vi "2 WaypointHeadingGoodness.vi"(3 "Waypoint Location":T1 {"North" format="%#_10f"; "East" format="%#_8f"}, 4 "Heading to Test":dbl) -> (1 "Goodness":dbl)   [LabVIEW 2011]
doc: "Takes the absolute wind vector, the heading of your next waypoint, and a test heading and outputs a goodness value for the test heading. The criteria is the speed to get to the waypoint.\n\nThe goodness is evaluated by taking the softmax of an angle with all possible complimenting angles (i.e. if the test heading is 10 degrees it is matched with -1 through -89; note that angles are adjusted to be degrees from directly at the waypoint). The specific calculation for finding the net velocity of a pair of angles requires the velocities from the polar plot."
uses:
  2 Typedefs/UTM Location.ctl
  2 Globals/2 Global.vi
  2 Globals/2 TuningConstants.vi
panel:
  out "Heading to Waypt":dbl
  # "Inputs"
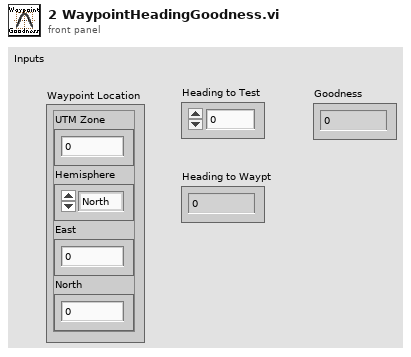
[diagram p1: front panel]
types:
  T1 = typedef "UTM Location.ctl" = cluster{"UTM Zone":dbl, "Hemisphere":enum16{"North", "South"}, "East":dbl, "North":dbl}
  T2 = typedef "Velocity.ctl" = cluster{"East":dbl, "North":dbl}
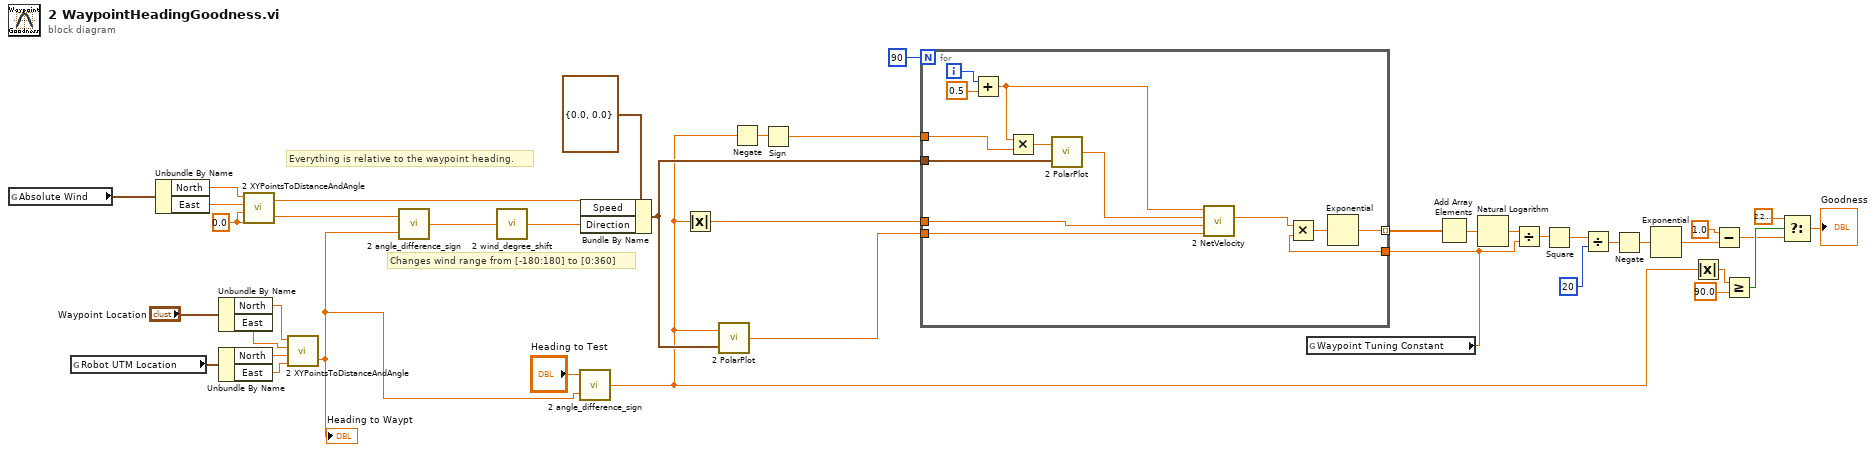
[diagram p0: block diagram]
diagram:
  w8 = 0.0
  # "Changes wind range from [-180:180] to [0:360]"
  # "Everything is relative to the waypoint heading."
  n1 = global read "2 Global.vi" "Absolute Wind"() -> (w11:T2)
  n2 = global read "2 Global.vi" "Robot UTM Location"() -> (w12:T1)
  n3 = Unbundle By Name(w11) -> ("North"=w9:dbl, "East"=w10:dbl)
  n4 = Unbundle By Name("Waypoint Location") -> ("North"=w21:dbl, "East"=w20:dbl)
  n5 = Unbundle By Name(w12) -> ("North"=w22:dbl, "East"=w23:dbl)
  n6 = call "2 XYPointsToDistanceAndAngle.vi"("East 2"=w8, "North 2"=w8, "East 1"=w10, "North 1"=w9) -> ("Angle Diff"=w25:dbl, "Distance"=w24:dbl)
  n7 = call "2 XYPointsToDistanceAndAngle.vi"("East 2"=w23, "North 2"=w22, "East 1"=w20, "North 1"=w21) -> ("Angle Diff"=w37:dbl)  [unwired: 1 out]
  "Heading to Waypt" <- w37
  n8 = call "2 angle_difference_sign.vi"("Angle 2"=w37, "Angle 1"=w25) -> ("Difference"=w41:dbl)
  n9 = call "2 wind_degree_shift.vi"("Wind Theta -180 - 180"=w41) -> ("Wind Theta 0-360"=w40:dbl)
  n10 = call "2 angle_difference_sign.vi"("Angle 2"=w37, "Angle 1"="Heading to Test") -> ("Difference"=w4:dbl)
  n11 = Bundle By Name(cluster=cluster{"Speed":dbl, "Direction":dbl} {"Speed"=0.0, "Direction"=0.0} ("input cluster"), "Speed"=w24, "Direction"=w40) -> (w27:cluster{"Speed":dbl, "Direction":dbl})
  n12 = Absolute Value(x=w4) -> (abs(x)=w2:dbl)
  n13 = call "2 PolarPlot.vi"("Wind Vector"=w27, "Boat Angle"=w4) -> ("Velocity"=w1:dbl)
  n14 = Negate(x=w4) -> (-x=w5:dbl)
  n15 = Sign(1:w5) -> (0:w6:dbl)
  n16 = global read "2 TuningConstants.vi" "Waypoint Tuning Constant"() -> (w3:dbl)
  n17 = for {
    N: 90 -> [_]
    tunnel: w27 -> [w54]
    tunnel: [w50] -> w13 mode=indexing
    tunnel: w6 -> [w43]
    tunnel: w3 -> [w45]
    tunnel: w2 -> [w47]
    tunnel: w1 -> [w46]
    i -> [w52]
    n18 = Add(x=w52, y=0.5) -> (x+y=w42:dbl)
    n19 = Multiply(x=w42, y=w43) -> (x*y=w53:dbl)
    n20 = call "2 PolarPlot.vi"("Wind Vector"=w54, "Boat Angle"=w53) -> ("Velocity"=w48:dbl)
    n21 = call "2 NetVelocity.vi"("Speed 2"=w46, "Angle 2"=w47, "Speed 1"=w48, "Angle 1"=w42) -> ("Net Velocity"=w44:dbl)  [unwired: 7 in]
    n22 = Multiply(x=w44, y=w45) -> (x*y=w49:dbl)
    n23 = Exponential(1:w49) -> (0:w50:dbl)
  }
  n24 = Add Array Elements(numeric array=w13) -> (sum=w16:dbl)
  n25 = Natural Logarithm(1:w16) -> (0:w15:dbl)
  n26 = Divide(x=w15, y=w3) -> (x/y=w14:dbl)
  n27 = Square(x=w14) -> (x^2=w17:dbl)
  n28 = Divide(x=w17, y=20) -> (x/y=w18:dbl)
  n29 = Negate(x=w18) -> (-x=w29:dbl)
  n30 = Exponential(1:w29) -> (0:w30:dbl)
  n31 = Absolute Value(x=w4) -> (abs(x)=w33:dbl)
  n32 = Subtract(x=1.0, y=w30) -> (x-y=w28:dbl)
  n33 = Greater Or Equal?(x=w33, y=90.0) -> (x >= y?=w35:bool)
  n34 = Select(t=2.220446049250313e-16, s=w35, f=w28) -> (s? t:f=→"Goodness":dbl)
